vi "Read with Trigger Model (Multiple Points).vi"(6 "Buffer Elements":u16(ring) items=["Date", "Extra", "Formatted", "Fractional", "Relative", "Seconds", "Status", "Time", "Timestamp", "Unit"], 8 "error in (no error)":errorcluster, 9 "Timeout (10000 ms)":i32=10000 format="%#.6g", 10 "Buffer Name":string="defbuffer1", 11 "VISA resource name":refnum<visa-resource-name>) -> (0 "error out":errorcluster, 1 "Element Value":string[](array[string]), 2 "Measurements":dbl[](array[numeric]), 3 "VISA resource name out":refnum<visa-resource-name>)   [LabVIEW 2018, in "Keithley DMM7512.lvlib"]
doc: "This VI starts the trigger model. Reads and returns multiple measurements from the instrument."
uses:
  <instrlib>/Keithley DMM7512/Keithley DMM7512.lvlib
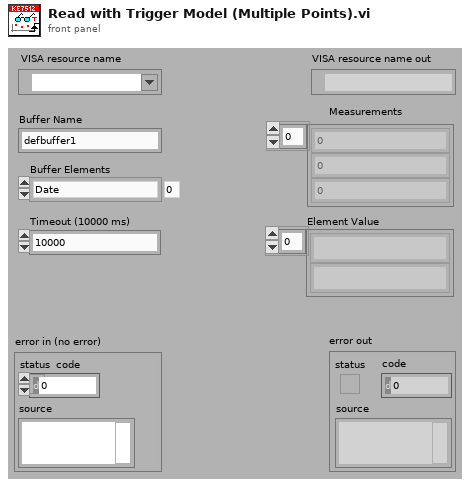
[diagram p1: front panel]
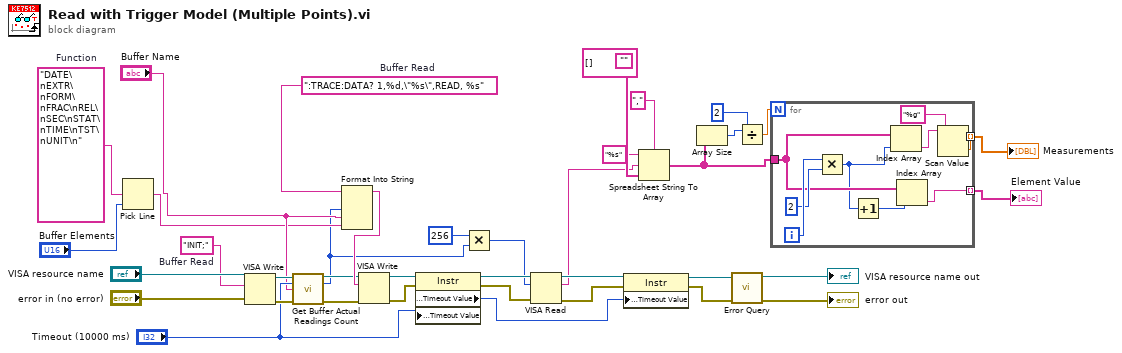
[diagram p0: block diagram]
diagram:
  w1 = "INIT;"  # Buffer Read
  (unwired) ""
  w24 = "DATE\nEXTR\nFORM\nFRAC\nREL\nSEC\nSTAT\nTIME\nTST\nUNIT\n"  # Function
  w27 = ":TRACE:DATA? 1,%d,\"%s\",READ, %s"  # Buffer Read
  n1 = Pick Line(multi-line string=w24, line index="Buffer Elements") -> (output string=w5:string)  [unwired: 1 out]
  n2 = VISA Write(VISA resource name="VISA resource name", write buffer=w1, error in (no error)="error in (no error)") -> (VISA resource name out=w11:refnum<visa-resource-name>, error out=w10:errorcluster)  [unwired: 1 out]
  n3 = call <instrlib>:"Get Buffer Actual Readings Count.vi"("VISA resource name"=w11, "Timeout (10000 ms)"="Timeout (10000 ms)", "Buffer Name (defbuffer1)"="Buffer Name", "error in (no error)"=w10) -> ("VISA resource name out"=w12:refnum<visa-resource-name>, "Actual Readings"=w3:i32, "error out"=w13:errorcluster)  [unwired: 9 in]
  n4 = Format Into String(format string=w27, w3, "Buffer Name", w5) -> (resulting string=w26:string)  [unwired: 2 in, 1 out]
  n5 = VISA Write(VISA resource name=w12, write buffer=w26, error in (no error)=w13) -> (VISA resource name out=w36:refnum<visa-resource-name>, error out=w35:errorcluster)  [unwired: 1 out]
  n6 = property class="Instr"(reference=w36, error in=w35, "General Settings:Timeout Value"="Timeout (10000 ms)") -> (reference out=w34:refnum<visa-resource-name>, error out=w33:errorcluster, "General Settings:Timeout Value"=w28:u32)
  n7 = Multiply(x=256, y=w3) -> (x*y=w4:i32)
  n8 = VISA Read(VISA resource name=w34, byte count=w4, error in (no error)=w33) -> (VISA resource name out=w32:refnum<visa-resource-name>, read buffer=w14:string, error out=w30:errorcluster)  [unwired: 1 out]
  n9 = property class="Instr"(reference=w32, error in=w30, "General Settings:Timeout Value"=w28) -> (reference out=w31:refnum<visa-resource-name>, error out=w29:errorcluster)
  n10 = Spreadsheet String To Array(delimiter (Tab)=",", format string="%s", spreadsheet string=w14, array type (2D Dbl)=string[] []) -> (array=w21:string[])
  n11 = Array Size(array=w21) -> (size(s)=w19:i32)
  n12 = call <instrlib>:"Error Query.vi"("error in (no error)"=w29, "VISA resource name"=w31) -> ("error out"=→"error out":errorcluster, "VISA resource name out"=→"VISA resource name out":refnum<visa-resource-name>)  [unwired: 6 in, 2 out]
  n13 = Divide(x=w19, y=2) -> (x/y=w17:dbl)
  n14 = for {
    N: w17 -> [_]
    tunnel: w21 -> [w45]
    tunnel: [w40] -> w16 mode=indexing
    tunnel: [w43] -> w15 mode=indexing
    i -> [w47]
    n15 = Multiply(x=w47, y=2) -> (x*y=w39:i32)
    n16 = Increment(x=w39) -> (x+1=w44:i32)
    n17 = Index Array(array=w45, index=w39) -> (element=w42:string)
    n18 = Index Array(array=w45, index=w44) -> (element=w43:string)
    n19 = Scan Value(string=w42, format string="%g") -> (value=w40:dbl)  [unwired: 1 in, 1 out]
  }
  "Measurements" <- w16
  "Element Value" <- w15
